vi "Get Pixel U16.vi"(8 "error in":errorcluster, 9 "col":i32, 10 "row":i32, 11 "Generic Image in":refnum<class "Generic Image.lvclass">) -> (0 "error out":errorcluster, 2 "Pixel":u16)   [LabVIEW 2024, in "Generic Image.lvclass"]
uses:
  Generic Image.lvclass
  Generic Image.lvclass/Generic Image.ctl
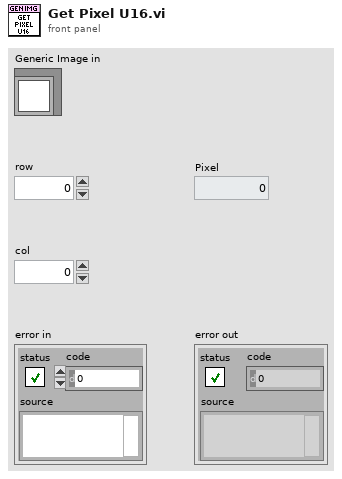
[diagram p1: front panel]
types:
  T1 = typedef "Generic Image.lvclass/Pixel Format.ctl" = enum16{"Grayscale (U8)", "Grayscale (I16)", "Grayscale (SGL)", "Complex (CSG)", "RGB (U32)", "HSL (U32)", "RGB (U64)", "Grayscale (U16)"}
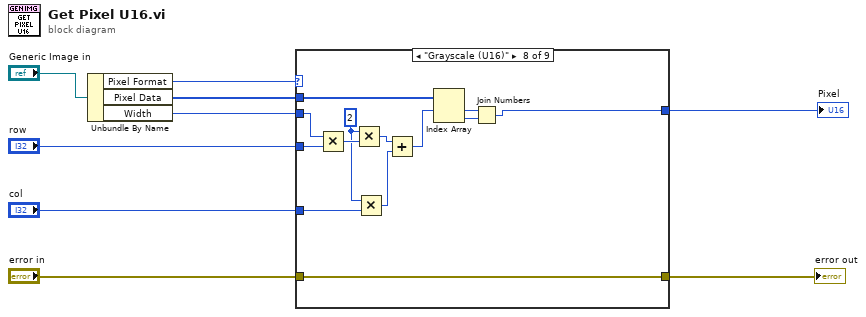
[diagram p0: block diagram]
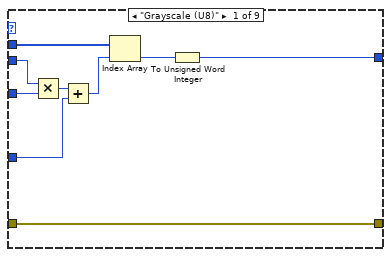
[diagram p2: hidden frame]
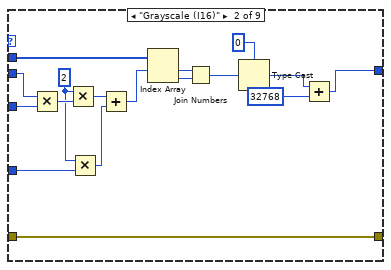
[diagram p3: hidden frame]
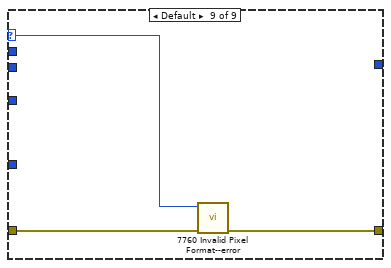
[diagram p9: hidden frame]
diagram:
  n1 = Unbundle By Name("Generic Image in") -> ("Pixel Format"=w8:T1, "Pixel Data"=w4:u8[], "Width"=w1:i32)
  n2 = case shown="\"Grayscale (U16)\"" w8 {
    selector: w8 -> [_ _ _ _ _ _ _ _ w54]
    tunnel: [w18 w34 _ _ _ _ _ w45 _] -> w5
    tunnel: "error in" -> [w17 w19 w36 w37 w38 w39 w40 w41 w56]
    tunnel: [w17 w19 w36 w37 w38 w39 w40 w41 w55] -> w6
    tunnel: w4 -> [w16 w26 _ _ _ _ _ w50 _]
    tunnel: "row" -> [w14 w24 _ _ _ _ _ w49 _]
    tunnel: "col" -> [w12 w25 _ _ _ _ _ w44 _]
    tunnel: w1 -> [w11 w23 _ _ _ _ _ w48 _]
    frame "Grayscale (U8)" {
      n3 = Multiply(x=w11, y=w14) -> (x*y=w13:i32)
      n4 = Add(x=w13, y=w12) -> (x+y=w10:i32)
      n5 = Index Array(array=w16, index=w10) -> (element=w15:u8)
      n6 = To Unsigned Word Integer(number=w15) -> (unsigned 16bit integer=w18:u16)
    }
    frame "Grayscale (I16)" {
      w28 = 2 ("x")
      n7 = Multiply(x=w23, y=w24) -> (x*y=w32:i32)
      n8 = Multiply(x=w28, y=w32) -> (x*y=w30:i32)
      n9 = Multiply(x=w28, y=w25) -> (x*y=w27:i32)
      n10 = Add(x=w30, y=w27) -> (x+y=w31:i32)
      n11 = Index Array(array=w26, index #1=w31) -> (element #1=w33:u8, element #2=w29:u8)  [unwired: 1 in]
      n12 = Join Numbers(hi=w33, lo=w29) -> ((hi.lo)=w22:u16)
      n13 = Type Cast(type=i16 0, x=w22) -> (*(type *) &x=w21:i16)
      n14 = Add(x=w21, y=u16 32768) -> (x+y=w34:u16)
    }
    frame "Grayscale (SGL)" {
    }
    frame "Complex (CSG)" {
    }
    frame "RGB (U32)" {
    }
    frame "HSL (U32)" {
    }
    frame "RGB (U64)" {
    }
    frame "Grayscale (U16)" {
      w43 = 2 ("x")
      n15 = Multiply(x=w48, y=w49) -> (x*y=w52:i32)
      n16 = Multiply(x=w43, y=w52) -> (x*y=w47:i32)
      n17 = Multiply(x=w43, y=w44) -> (x*y=w42:i32)
      n18 = Add(x=w47, y=w42) -> (x+y=w51:i32)
      n19 = Index Array(array=w50, index #1=w51) -> (element #1=w53:u8, element #2=w46:u8)  [unwired: 1 in]
      n20 = Join Numbers(hi=w53, lo=w46) -> ((hi.lo)=w45:u16)
    }
    frame Default {
      n21 = call "7760 Invalid Pixel Format--error.vi"("error in"=w56, "Argument"=w54) -> ("error out"=w55:errorcluster)  [unwired: 9 in]
    }
  }
  "error out" <- w6
  "Pixel" <- w5
